vi "Wait Rendezvous.vi"(8 "error in (no error)":errorcluster, 9 "Timeout":i32=-1, 10 "Rendezvous Index":i32, 11 "System Actor in":refnum<class "System Actor.lvclass">) -> (0 "error out":errorcluster, 1 "Timeout?":bool, 3 "System Actor out":refnum<class "System Actor.lvclass">)   [LabVIEW 2024, in "System Actor.lvclass"]
uses:
  System Actor.lvclass
  System Actor.lvclass/System Actor.ctl
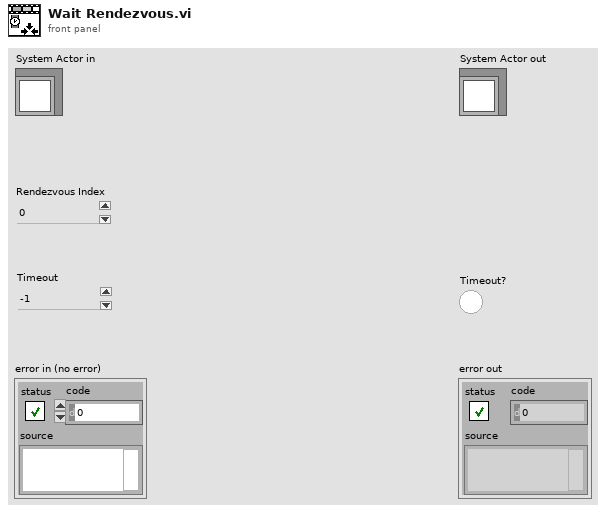
[diagram p1: front panel]
types:
  T1 = typedef "Rendezvous RefNum" = refnum<k1>
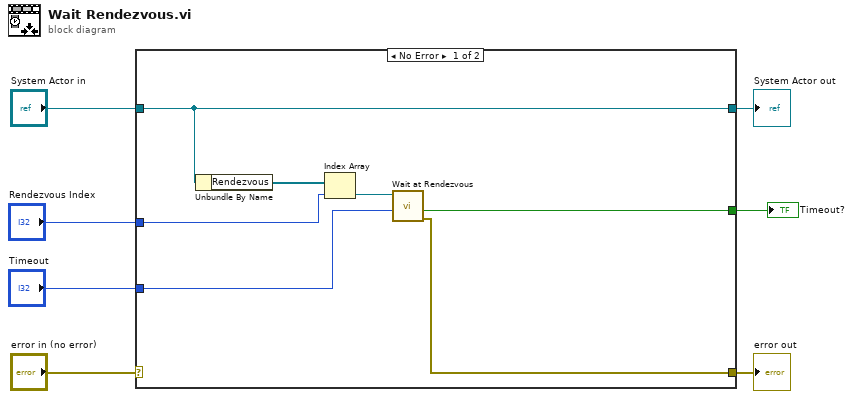
[diagram p0: block diagram]
diagram:
  n1 = case shown="No Error" "error in (no error)" {
    selector: "error in (no error)" -> [_ w16]
    tunnel: [w9 w16] -> w6
    tunnel: [w14 w15] -> w4
    tunnel: "System Actor in" -> [w14 w15]
    tunnel: "Rendezvous Index" -> [w12 _]
    tunnel: "Timeout" -> [w10 _]
    tunnel: [w8 _] -> w1
    frame No Error {
      n2 = Unbundle By Name(w14) -> ("Rendezvous"=w13:T1[])
      n3 = Index Array(array=w13, index=w12) -> (element=w11:T1)
      n4 = call <vilib>:"Wait at Rendezvous.vi"("ms timeout (-1)"=w10, "rendezvous"=w11) -> ("error out"=w9:errorcluster, "timed out"=w8:bool)  [unwired: 3 in, 1 out]
    }
    frame Error {
    }
  }
  "error out" <- w6
  "System Actor out" <- w4
  "Timeout?" <- w1
